vi "Config has been set.vi"(0 "Type Signal":T1={"DAQ Board Name"="DAQ_Simu1", "Analogicos Canales"=["DAQ_Simu1/ai1", "DAQ_Simu1/ai2"], "Port Digitales"=[], "Tiempo"=100.0, "number of samples "=1000, "rate"=1000.0, "Type"=enum."Analogico"}, 1 "Nombre de la Prueba":string, 3 "error in":errorcluster) -> (10 "error out":errorcluster)   [LabVIEW 2020, in "Settings.lvlib"]
doc: "Config has been set in the table\n_____\nCreated using Delacor QMH Event Scripter 6.0.0.121."
uses:
  Settings.lvlib
  typeSignal--cluster.ctl
  Config has been set Argument--cluster.ctl
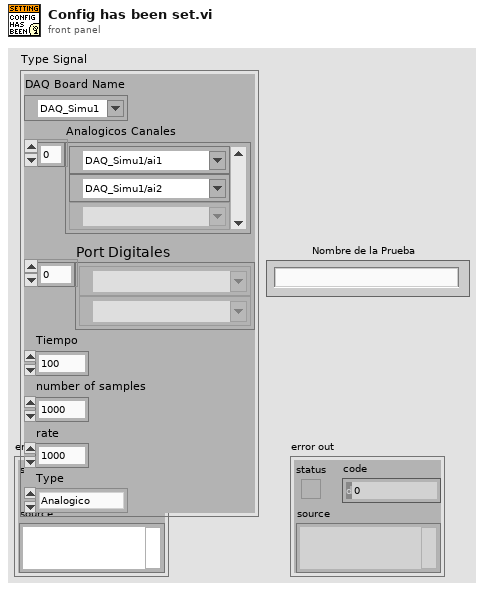
[diagram p1: front panel]
types:
  T1 = typedef "typeSignal--cluster.ctl" = cluster{"DAQ Board Name":tag, "Analogicos Canales":tag[], "Port Digitales":tag[], "Tiempo":dbl, "number of samples ":i32, "rate":dbl, "Type":enum16{"Analogico", "Digital"}}
  T2 = typedef "Settings.lvlib/Config has been set Argument--cluster.ctl" = cluster{"Nombre de la Prueba":string, "Type Signal":T1}
  T3 = typedef "Settings.lvlib/Broadcast Events--cluster.ctl" = cluster{"Module Did Init":refnum<user-event>, "Status Updated":refnum<user-event>, "Error Reported":refnum<user-event>, "Module Did Stop":refnum<user-event>, "Update Module Execution Status":refnum<user-event>, "Config has been set":refnum<user-event>}
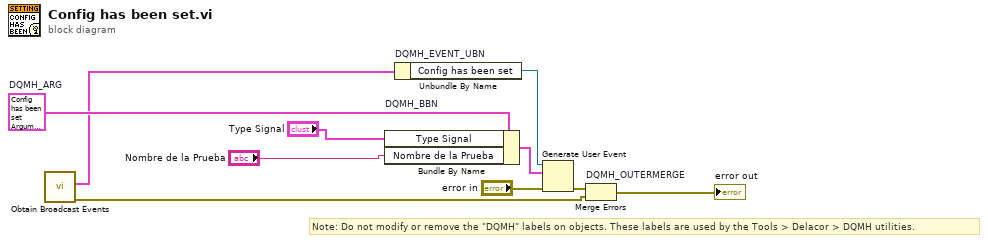
[diagram p0: block diagram]
diagram:
  w5 = T2 {"Nombre de la Prueba"="", "Type Signal"={"DAQ Board Name"="DAQ_Simu1", "Analogicos Canales"=["DAQ_Simu1/ai1", "DAQ_Simu1/ai2"], "Port Digitales"=[], "Tiempo"=100.0, "number of samples "=1000, "rate"=1000.0, "Type"=enum."Analogico"}}  # DQMH_ARG
  # "Note: Do not modify or remove the \"DQMH\" labels on objects. These labels are used by the Tools > Delacor > DQMH utilities."
  n1 = call "Obtain Broadcast Events.vi"() -> ("error out"=w4:errorcluster, "Settings Broadcast Events"=w3:T3)  [unwired: 10 in]
  n2 = Bundle By Name "DQMH_BBN"(cluster=w5, "Type Signal"="Type Signal", "Nombre de la Prueba"="Nombre de la Prueba") -> (w8:T2)
  n3 = Unbundle By Name "DQMH_EVENT_UBN"(w3) -> ("Config has been set"=w7:refnum<user-event>)
  n4 = Generate User Event(user event=w7, event data cluster=w8, error in="error in") -> (error out=w6:errorcluster)  [unwired: 1 in, 1 out]
  n5 = Merge Errors "DQMH_OUTERMERGE"(w6, w4) -> (→"error out":errorcluster)
